vi "Flush Buffer.vi"(8 "error in (no error)":errorcluster, 11 "2D U16 Group With ID DVR Queue in":refnum<class "2D U16 Group With ID DVR Queue.lvclass">) -> (0 "error out":errorcluster, 3 "2D U16 Group With ID DVR Queue out":refnum<class "2D U16 Group With ID DVR Queue.lvclass">)   [LabVIEW 2024, in "2D U16 Group With ID DVR Queue.lvclass"]
uses:
  2D U16 Group With ID DVR Queue.lvclass
  2D U16 Group With ID DVR Queue.lvclass/2D U16 Group With ID DVR Queue.ctl
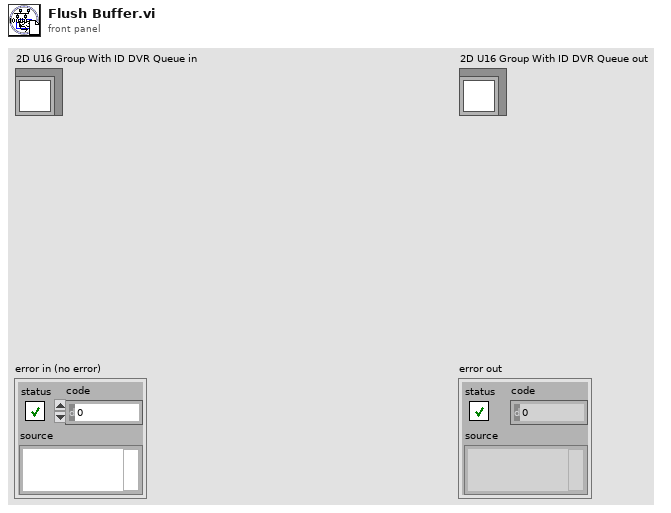
[diagram p1: front panel]
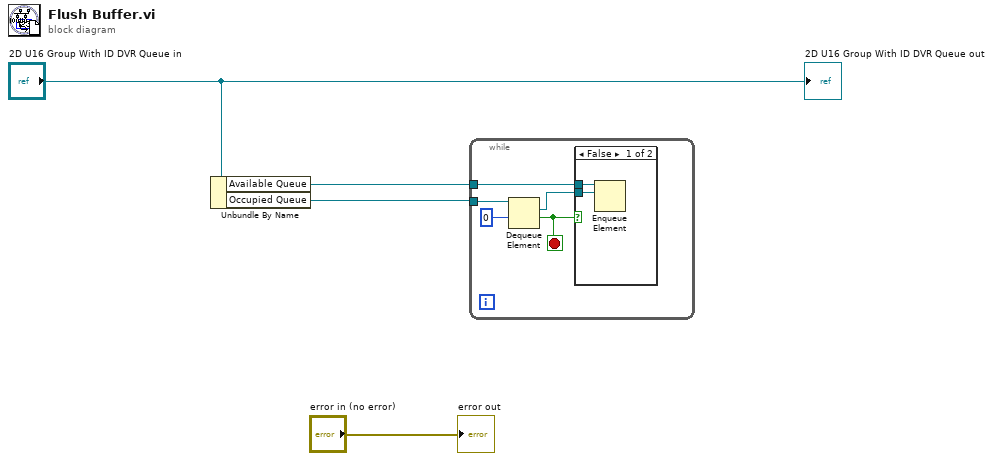
[diagram p0: block diagram]
diagram:
  n1 = Unbundle By Name("2D U16 Group With ID DVR Queue in") -> ("Available Queue"=w2:refnum<queue>, "Occupied Queue"=w1:refnum<queue>)
  n2 = while {
    tunnel: w1 -> [w9]
    tunnel: w2 -> [w7]
    stop <- w5 stop-if-true
    n3 = Dequeue Element(queue=w9, timeout in ms (-1)=0) -> (element=w6:refnum<data-value>, timed out?=w5:bool)  [unwired: 1 in, 2 out]
    n4 = case shown="False" w5 {
      tunnel: w7 -> [w11 _]
      tunnel: w6 -> [w10 _]
      frame False {
        n5 = Enqueue Element(queue=w11, element=w10) -> ()  [unwired: 2 in, 3 out]
      }
      frame True {
      }
    }
  }
  "error out" <- "error in (no error)"
  "2D U16 Group With ID DVR Queue out" <- "2D U16 Group With ID DVR Queue in"
